vi "Enque(MoveToPosition).vi"(5 "Message Command":string="StartAbsMove", 6 "Polarization":u16(ring) items=["Vertical", "Horizontal"], 7 "at front (F)":bool, 8 "error in":errorcluster, 9 "TR Module/Raster num":i32, 10 "Position":T1, 11 "Message que":T2) -> (0 "error out":errorcluster, 3 "Message que out":T2)   [LabVIEW 2017]
doc: "Transmit a message with a DBL array payload.\nFor a regular message, enqueue the message. For a priority message, enqueue it at the front of the queue.\n\nBolder Software LLC"
uses:
  MessageQue/MessageQue.ctl
  MessageQue/MessageCluster.ctl
  MoveAllAbsolute.ctl
  MessageQue/MessageQue.lvlib
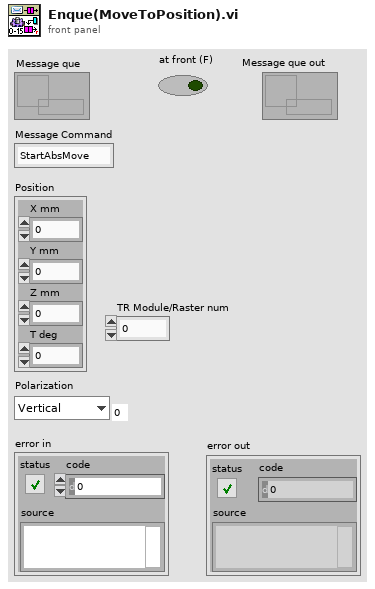
[diagram p1: front panel]
types:
  T1 = cluster{"X mm":dbl, "Y mm":dbl, "Z mm":dbl, "T deg":dbl}
  T2 = typedef "MessageQue.lvlib/MessageQue.ctl" = refnum<queue>
  T3 = typedef "MoveAllAbsolute.ctl" = cluster{"MoveType":string, "Move Params":dbl[]}
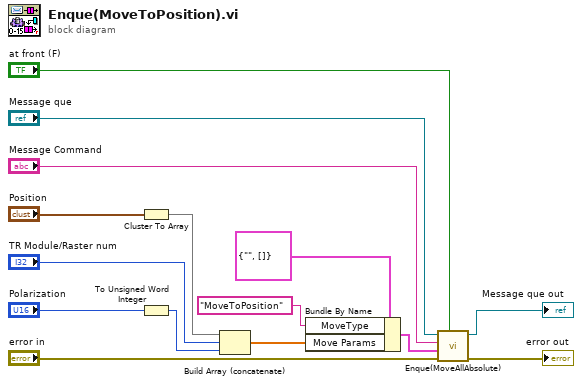
[diagram p0: block diagram]
diagram:
  n1 = Cluster To Array(cluster="Position") -> (array=w3:dbl[])
  n2 = To Unsigned Word Integer(number="Polarization") -> (unsigned 16bit integer=w2:u16)
  n3 = Build Array (concatenate)(w3, "TR Module/Raster num", w2) -> (w11:dbl[])
  n4 = Bundle By Name(cluster=T3 {"MoveType"="", "Move Params"=[]} ("Message Payload  array"), "MoveType"="MoveToPosition", "Move Params"=w11) -> (w13:T3)
  n5 = call "Enque(MoveAllAbsolute).vi"("at front (F)"="at front (F)", "error in"="error in", "Message Payload  array"=w13, "Message Command"="Message Command", "Message que"="Message que") -> ("error out"=→"error out":errorcluster, "Message que out"=→"Message que out":T2)  [unwired: 5 in]
